vi "GetState_Available.vi"(8 "error in (no error)":errorcluster caption="错误输入（无错误）", 11 "TCPClientClass输入":refnum<class "TCPClientClass.lvclass">) -> (0 "error out":errorcluster caption="错误输出", 2 "可用？":bool, 3 "TCPClientClass输出":refnum<class "TCPClientClass.lvclass">)   [LabVIEW 2019, in "TCPClientClass.lvclass"]
uses:
  TCPClientClass.lvclass
  TCPClientClass.lvclass/TCPClientClass.ctl
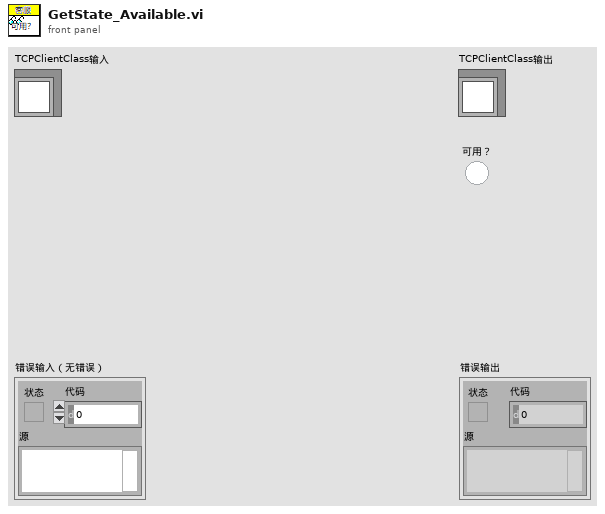
[diagram p1: front panel]
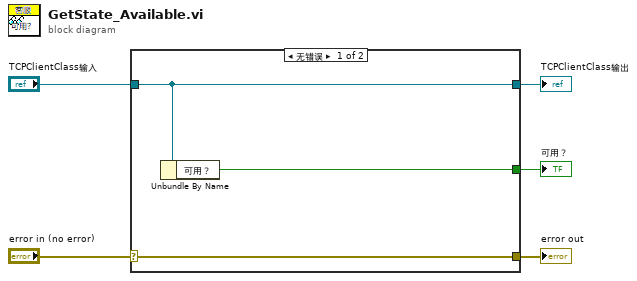
[diagram p0: block diagram]
diagram:
  n1 = case shown="无错误" "error in (no error)" {
    selector: "error in (no error)" -> [w8 w9]
    tunnel: [w8 w9] -> w4
    tunnel: [w7 w10] -> w2
    tunnel: "TCPClientClass输入" -> [w7 w10]
    tunnel: [w6 _] -> w1
    frame No Error {
      n2 = Unbundle By Name(w7) -> ("可用？"=w6:bool)
    }
    frame Error {
    }
  }
  "error out" <- w4
  "TCPClientClass输出" <- w2
  "可用？" <- w1
